vi "Swerve Drive.vi"(0 "X":dbl, 1 "Rot. Point X":dbl, 3 "Rot. Point Y":dbl, 5 "Y":dbl, 7 "Z":dbl, 11 "Error In":errorcluster, 12 "Robot Centric?":bool=TRUE, 13 "Autonomous?":bool, 14 "Yaw":dbl) -> (4 "Front Left Output":dbl, 6 "Front Right Output":dbl, 8 "Back Left Output":dbl, 10 "Back Right Output":dbl, 15 "Error Out":errorcluster)   [LabVIEW 2017]
uses:
  Public/Documents/Cross The Road Electronics/Phoenix-LabVIEW/Motor Controller/Controls/CTRE_Phoenix_MotorControl_ControlMode.ctl
  <vilib>/Rock Robotics/Network Tables/NT Read Number.vi
  <vilib>/Rock Robotics/Network Tables/NT Write Numeric Array.vi
panel:
  in  "Robot Length":dbl=33.5
  in  "Robot Width":dbl=28.5
  # "Swerve Drive Teleoperated Control\nFRC Team 34"
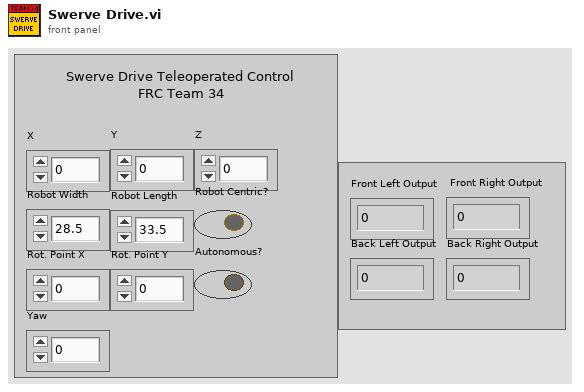
[diagram p1: front panel]
types:
  T1 = typedef "CTRE_Phoenix_MotorControl_ControlMode.ctl" = u16
  T2 = enum16{"Front Left", "Front Right", "Back Left", "Back Right"}
  T3 = typedef "WPI_MotorControlDeviceRef.ctl" = cluster{"DeviceStatus":errorcluster, "Type":T4, "PWM":cluster{"PWM Channel":T5, "DeadBand":T6}, "CAN":cluster{"Device Number":u8, "SetOutput VI Ref":variant, "GetOutput VI Ref":variant, "Enable VI Ref":variant, "Disable VI Ref":variant, "Data":variant}, "Invert":bool, "DIO PWM":cluster{"PWM \"Enable\" Channel":T5, "DIOChannel":T7, "PWM Rate":dbl}}
  T4 = typedef "WPI_MotorControlType.ctl" = enum16{"PWM", "CAN", "DIO PWM"}
  T5 = typedef "FPGA_DIOPWMChannel.ctl" = enum8{"PWM 0", "PWM 1", "PWM 2", "PWM 3", "PWM 4", "PWM 5", "PWM 6", "PWM 7", "PWM 8", "PWM 9", "PWM MXP 0", "PWM MXP 1", "PWM MXP 2", "PWM MXP 3", "PWM MXP 4", "PWM MXP 5", "PWM MXP 6", "PWM MXP 7", "PWM MXP 8", "PWM MXP 9", "Invalid"}
  T6 = typedef "WPI_PWMDeadband.ctl" = cluster{"Name":string, "maxPositivePwm":i32, "minPositivePwm":i32, "centerPwm":i32, "maxNegativePwm":i32, "minNegativePwm":i32, "angularRange":u16}
  T7 = typedef "FPGA_DIOChannel.ctl" = enum8{"DIO 0", "DIO 1", "DIO 2", "DIO 3", "DIO 4", "DIO 5", "DIO 6", "DIO 7", "DIO 8", "DIO 9", "DIO MXP 0", "DIO MXP 1", "DIO MXP 2", "DIO MXP 3", "DIO MXP 4", "DIO MXP 5", "DIO MXP 6", "DIO MXP 7", "DIO MXP 8", "DIO MXP 9", "DIO MXP 10", "DIO MXP 11", "DIO MXP 12", "DIO MXP 13", "DIO MXP 14", "DIO MXP 15", "SPI Port CS1", "SPI Port CS2", "SPI Port CS3", "SPI Port MISO", "SPI Port MOSI", "Invalid"}
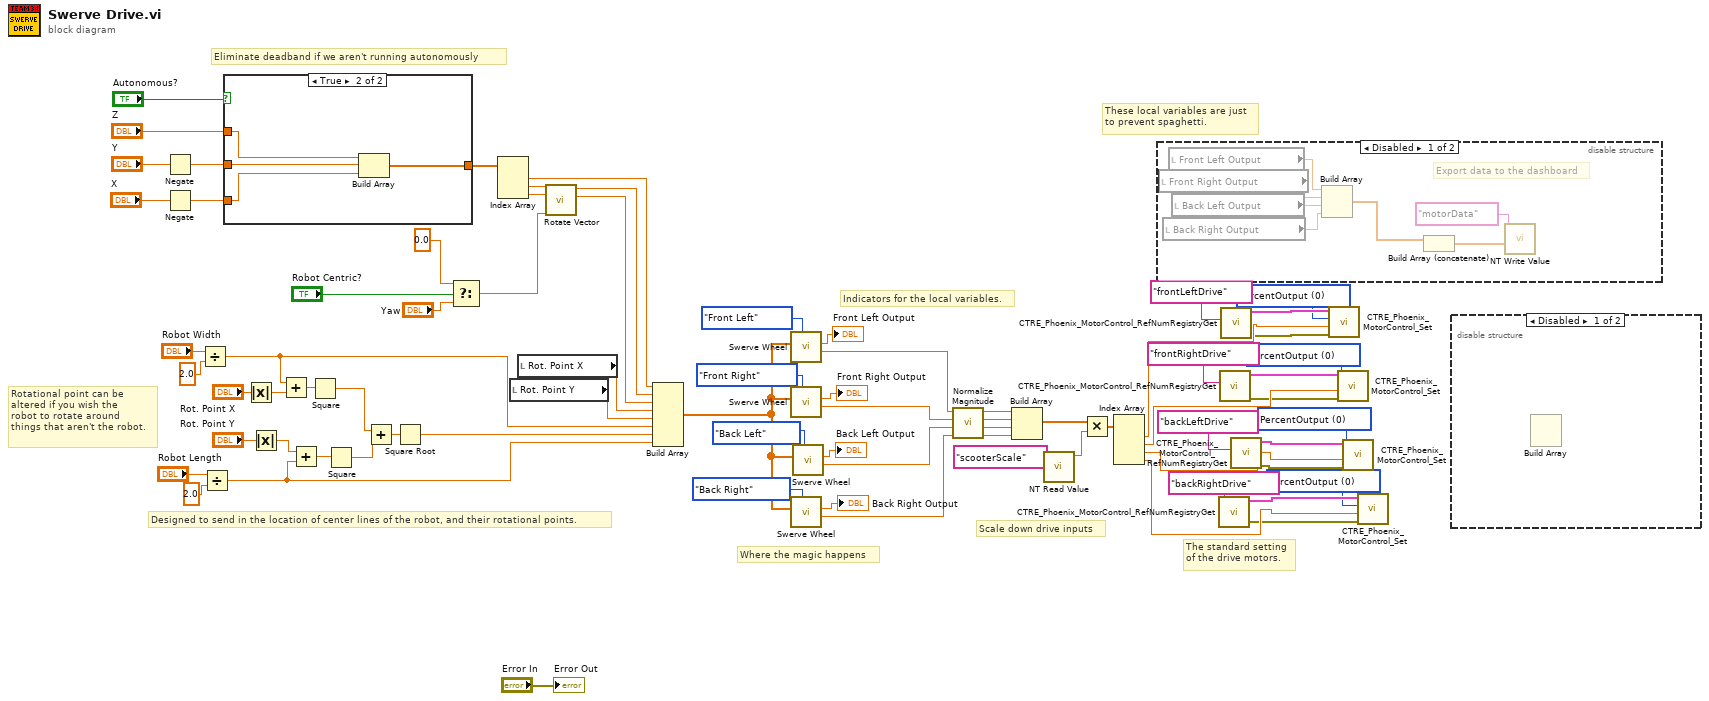
[diagram p0: block diagram]
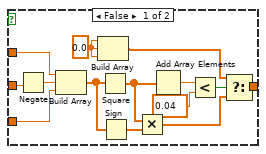
[diagram p4: hidden frame]
diagram:
  w1 = T1 0 items=["PercentOutput"=0, "Position"=1, "Velocity"=2, "Current"=3, "Follower"=5, "MotionProfile"=6, "MotionMagic"=7, "MotionMagicArc"=8, "MotionProfileArc"=10, "Disabled"=15] ("Control Mode")
  w2 = T1 0 items=["PercentOutput"=0, "Position"=1, "Velocity"=2, "Current"=3, "Follower"=5, "MotionProfile"=6, "MotionMagic"=7, "MotionMagicArc"=8, "MotionProfileArc"=10, "Disabled"=15] ("Control Mode")
  w3 = T1 0 items=["PercentOutput"=0, "Position"=1, "Velocity"=2, "Current"=3, "Follower"=5, "MotionProfile"=6, "MotionMagic"=7, "MotionMagicArc"=8, "MotionProfileArc"=10, "Disabled"=15] ("Control Mode")
  w4 = T1 0 items=["PercentOutput"=0, "Position"=1, "Velocity"=2, "Current"=3, "Follower"=5, "MotionProfile"=6, "MotionMagic"=7, "MotionMagicArc"=8, "MotionProfileArc"=10, "Disabled"=15] ("Control Mode")
  # "Indicators for the local variables."
  # "Rotational point can be \naltered if you wish the \nrobot to rotate around \nthings that aren't the robot."
  # "Scale down drive inputs"
  # "Eliminate deadband if we aren't running autonomously"
  # "These local variables are just \nto prevent spaghetti."
  # "Where the magic happens"
  # "The standard setting\nof the drive motors."
  # "Designed to send in the location of center lines of the robot, and their rotational points."
  n1 = Negate(x="Y") -> (-x=w22:dbl)
  n2 = Negate(x="X") -> (-x=w21:dbl)
  n3 = Divide(x="Robot Width", y=2.0) -> (x/y=w49:dbl)
  n4 = Divide(x="Robot Length", y=2.0) -> (x/y=w47:dbl)
  n5 = case shown="True" "Autonomous?" {
    tunnel: w22 -> [w80 w93]
    tunnel: [w79 w91] -> w75
    tunnel: "Z" -> [w78 w94]
    tunnel: w21 -> [w77 w92]
    frame False {
      w86 = 0.0 ("element")
      n6 = Negate(x=w80) -> (-x=w82:dbl)
      n7 = Build Array(w78, w82, w77) -> (w85:dbl[])
      n8 = Build Array(w86, w86, w86) -> (w87:dbl[])
      n9 = Square(x=w85) -> (x^2=w83:dbl[])
      n10 = Sign(1:w85) -> (0:w84:dbl[])
      n11 = Multiply(x=w83, y=w84) -> (x*y=w81:dbl[])
      n12 = Add Array Elements(numeric array=w83) -> (sum=w90:dbl)
      n13 = Less?(x=w90, y=0.04 ("x")) -> (x < y?=w88:bool)
      n14 = Select(t=w87, s=w88, f=w81) -> (s? t:f=w79:dbl[])
    }
    frame True {
      n15 = Build Array(w94, w93, w92) -> (w91:dbl[])
    }
  }
  n16 = Absolute Value(x="Rot. Point X") -> (abs(x)=w61:dbl)
  n17 = Absolute Value(x="Rot. Point Y") -> (abs(x)=w58:dbl)
  n18 = Add(x=w49, y=w61) -> (x+y=w60:dbl)
  n19 = Add(x=w58, y=w47) -> (x+y=w59:dbl)
  n20 = Square(x=w60) -> (x^2=w56:dbl)
  n21 = Square(x=w59) -> (x^2=w57:dbl)
  n22 = Add(x=w56, y=w57) -> (x+y=w55:dbl)
  n23 = Square Root(x=w55) -> (sqrt(x)=w48:dbl)
  n24 = Select(t=0.0, s="Robot Centric?", f="Yaw") -> (s? t:f=w68:dbl)
  n25 = Index Array(array=w75) -> (element #1=w54:dbl, element #2=w70:dbl, element #3=w69:dbl)  [unwired: 3 in]
  n26 = local read "Rot. Point Y"() -> (w50:dbl)
  n27 = local read "Rot. Point X"() -> (w51:dbl)
  n28 = call "Rotate Vector.vi"("Angle"=w68, "X"=w69, "Y"=w70) -> ("X'"=w52:dbl, "Y'"=w53:dbl)  [unwired: 7 in]
  n29 = Build Array(w54, w53, w52, w51, w50, w49, w48, w47) -> (w46:dbl[])
  n30 = call "Swerve Wheel.vi"("Wheel"=T2."Front Left", "Inputs"=w46) -> ("Speed"=w41:dbl, "Motor Output"=→"Front Left Output":dbl)  [unwired: 8 in]
  n31 = call "Swerve Wheel.vi"("Wheel"=T2."Front Right", "Inputs"=w46) -> ("Speed"=w40:dbl, "Motor Output"=→"Front Right Output":dbl)  [unwired: 8 in]
  n32 = call "Swerve Wheel.vi"("Wheel"=T2."Back Right", "Inputs"=w46) -> ("Speed"=w38:dbl, "Motor Output"=→"Back Right Output":dbl)  [unwired: 8 in]
  n33 = call "Swerve Wheel.vi"("Wheel"=T2."Back Left", "Inputs"=w46) -> ("Speed"=w39:dbl, "Motor Output"=→"Back Left Output":dbl)  [unwired: 8 in]
  n34 = call "Normalize Magnitude.vi"("D"=w38, "C"=w39, "B"=w40, "A"=w41) -> ("D'"=w34:dbl, "C'"=w35:dbl, "B'"=w36:dbl, "A'"=w37:dbl)  [unwired: 4 in]
  n35 = Build Array(w37, w36, w35, w34) -> (w33:dbl[])
  n36 = call-poly <vilib>:"NT Read Value.vi"("Name"="scooterScale") -> ("Numeric"=w31:dbl)  [unwired: 9 in, 1 out]
  n37 = Multiply(x=w33, y=w31) -> (x*y=w30:dbl[])
  n38 = Index Array(array=w30) -> (element #1=w15:dbl, element #2=w9:dbl, element #3=w6:dbl, element #4=w12:dbl)  [unwired: 4 in]
  n39 = disable-structure shown="Disabled" {
    frame Disabled {
      # "Export data to the dashboard"
      n40 = local read "Front Right Output"() -> (w97:dbl)
      n41 = local read "Back Right Output"() -> (w95:dbl)
      n42 = local read "Front Left Output"() -> (w98:dbl)
      n43 = local read "Back Left Output"() -> (w96:dbl)
      n44 = Build Array(w98, w97, w96, w95) -> (w101:dbl[])
      n45 = Build Array (concatenate)(w101) -> (w100:dbl[])  [unwired: 1 in]
      n46 = call-poly <vilib>:"NT Write Value.vi"("Numeric Array"=w100, "Name"="motorData") -> ()  [unwired: 9 in, 1 out]
    }
    frame Enabled {
    }
  }
  n47 = call "CTRE_Phoenix_MotorControl_RefNumRegistryGet.vi"("refnum name"="backRightDrive") -> ("error out"=w11:errorcluster, "PhoenixMotorControlDevRef"=w13:T3)  [unwired: 9 in]
  n48 = call "CTRE_Phoenix_MotorControl_RefNumRegistryGet.vi"("refnum name"="frontRightDrive") -> ("error out"=w8:errorcluster, "PhoenixMotorControlDevRef"=w10:T3)  [unwired: 9 in]
  n49 = call "CTRE_Phoenix_MotorControl_RefNumRegistryGet.vi"("refnum name"="frontLeftDrive") -> ("error out"=w14:errorcluster, "PhoenixMotorControlDevRef"=w16:T3)  [unwired: 9 in]
  n50 = call "CTRE_Phoenix_MotorControl_RefNumRegistryGet.vi"("refnum name"="backLeftDrive") -> ("error out"=w5:errorcluster, "PhoenixMotorControlDevRef"=w7:T3)  [unwired: 9 in]
  n51 = call "CTRE_Phoenix_MotorControl_Set.vi"("error in (no error)"=w14, "Output"=w15, "Control Mode"=w4, "PhoenixMotorControlDevRef"=w16) -> ()  [unwired: 5 in, 3 out]
  n52 = call "CTRE_Phoenix_MotorControl_Set.vi"("error in (no error)"=w8, "Output"=w9, "Control Mode"=w3, "PhoenixMotorControlDevRef"=w10) -> ()  [unwired: 5 in, 3 out]
  n53 = call "CTRE_Phoenix_MotorControl_Set.vi"("error in (no error)"=w5, "Output"=w6, "Control Mode"=w2, "PhoenixMotorControlDevRef"=w7) -> ()  [unwired: 5 in, 3 out]
  n54 = call "CTRE_Phoenix_MotorControl_Set.vi"("error in (no error)"=w11, "Output"=w12, "Control Mode"=w1, "PhoenixMotorControlDevRef"=w13) -> ()  [unwired: 5 in, 3 out]
  n55 = disable-structure shown="Disabled" {
    frame Disabled {
      n56 = Build Array() -> (w102:void[], w106:dbl, w105:dbl, w104:dbl, w103:dbl)
    }
    frame Enabled {
    }
  }
  "Error Out" <- "Error In"
